vi "N6705B_DIG_OUT.vi"(8 "error in (no error)":errorcluster {"code" format="%.0x"}, 10 "DUT_1_4":i32=2, 11 "VISA Refnum in":refnum<visa-resource-name>="VAL_N6705B") -> (0 "error out":errorcluster {"code" format="%.0x"}, 3 "VISA Refnum out":refnum<visa-resource-name>)   [LabVIEW 2015]
uses:
  <instrlib>/Agilent N6700 Series/Agilent N6700 Series.lvlib
panel:
  out "number":u32
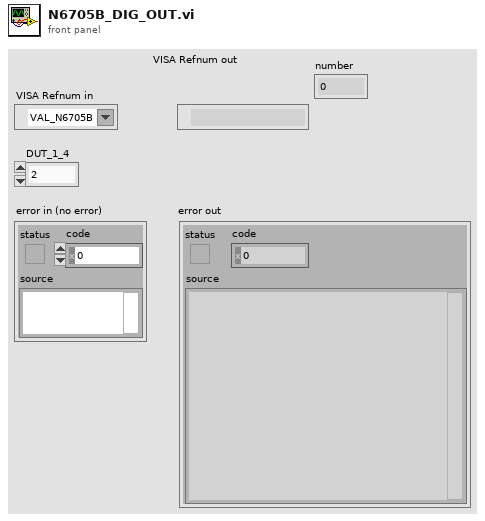
[diagram p1: front panel]
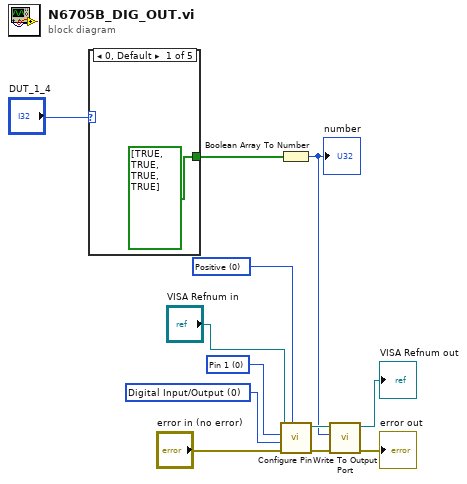
[diagram p0: block diagram]
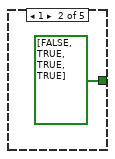
[diagram p2: hidden frame]
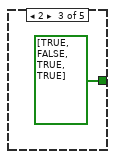
[diagram p3: hidden frame]
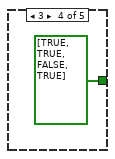
[diagram p4: hidden frame]
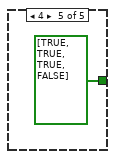
[diagram p5: hidden frame]
diagram:
  w8 = 0 items=["Positive", "Negative"] ("Polarity (0: Positive)")
  w9 = 0 items=["Digital Input/Output", "Digital Input-only", "Trigger Output", "Trigger Input", "Fault", "Inhibit"] ("Pin Function (0: Digital Input/Output)")
  w7 = u16 0 items=["Pin 1", "Pin 2", "Pin 3"] ("Pin Name (0: Pin 1)")
  n1 = case shown="0, Default" "DUT_1_4" {
    tunnel: [bool[] [TRUE, TRUE, TRUE, TRUE] bool[] [FALSE, TRUE, TRUE, TRUE] bool[] [TRUE, FALSE, TRUE, TRUE] bool[] [TRUE, TRUE, FALSE, TRUE] bool[] [TRUE, TRUE, TRUE, FALSE]] -> w4
    frame 0, Default {
    }
    frame 1 {
    }
    frame 2 {
    }
    frame 3 {
    }
    frame 4 {
    }
  }
  n2 = Boolean Array To Number(Boolean array=w4) -> (number=w3:u32)
  "number" <- w3
  n3 = call <instrlib>:"Configure Pin.vi"("Polarity (0: Positive)"=w8, "error in (no error)"="error in (no error)", "Pin Function (0: Digital Input/Output)"=w9, "Pin Name (0: Pin 1)"=w7, "VISA resource name"="VISA Refnum in") -> ("error out"=w6:errorcluster, "VISA resource name out"=w5:refnum<visa-resource-name>)  [unwired: 5 in]
  n4 = call <instrlib>:"Write To Output Port.vi"("error in (no error)"=w6, "Data (7)"=w3, "VISA resource name"=w5) -> ("error out"=→"error out":errorcluster, "VISA resource name out"=→"VISA Refnum out":refnum<visa-resource-name>)  [unwired: 7 in]
